vi "扭矩.vi"() -> ()   [LabVIEW 2020]
uses:
  <userlib>/DAQNavi Polymorphic VI/create/DAQNavi Create Channel(AI-Voltage).vi
  Global_Variable/Global.vi
  Global_Variable/A131258.vi
  <userlib>/DAQNavi Polymorphic VI/read/DAQNavi Read (Analog 1D DBL NChan 1Samp).vi
  <userlib>/_MGI/1D Array/MGI Running Average/MGI Running Average(DBL).vi
  <vilib>/ptbypt/NI_PtbyPt.lvlib
panel:
  out "左加载":dbl
  out "右加载":dbl
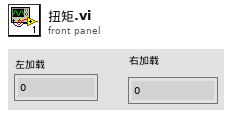
[diagram p1: front panel]
types:
  T1 = cluster{"左平均扭矩":cluster{"正转":dbl, "反转":dbl}, "左矩波动":cluster{"正转":dbl, "反转":dbl}, "左空载":cluster{"正转":dbl, "反转":dbl}, "右平均扭矩":cluster{"正转":dbl, "反转":dbl}, "右扭矩波动":cluster{"正转":dbl, "反转":dbl}, "右空载":cluster{"正转":dbl, "反转":dbl}, "扭矩对称":cluster{"左":dbl, "右":dbl}, "左零点漂移":cluster{"正":dbl, "反":dbl}, "右零点漂移":cluster{"正":dbl, "反":dbl}}
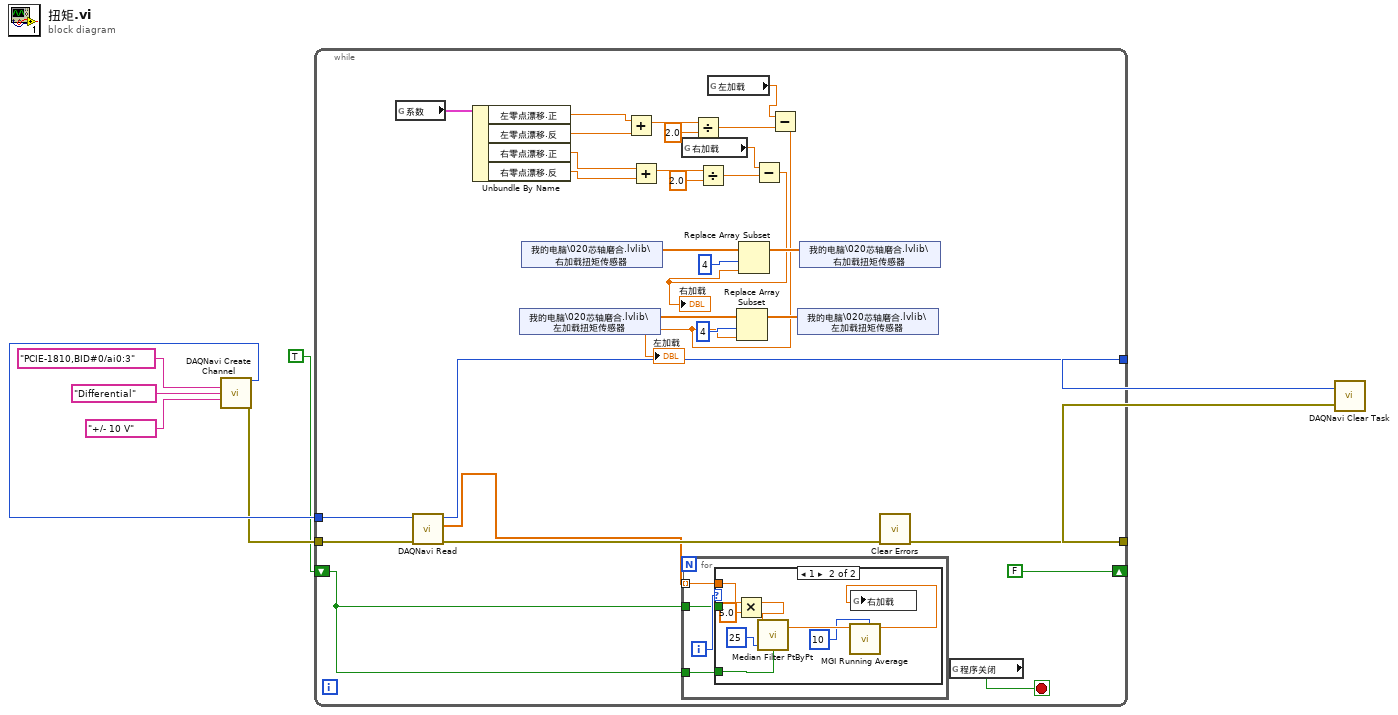
[diagram p0: block diagram]
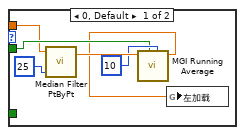
[diagram p2: hidden frame]
diagram:
  n1 = call-poly <userlib>:"DAQNavi Create Channel.vi"("physical channels"="PCIE-1810,BID#0/ai0:3", "signal type"="Differential", "value range"="+/- 10 V") -> ("task out"=w6:i32, "error out"=w5:errorcluster)  [unwired: 11 in]
  n2 = while {
    tunnel: w6 -> [w38]
    tunnel: w5 -> [w37]
    tunnel: [w33] -> w3
    tunnel: [w34] -> w2
    shift-right: [FALSE] -> _
    shift-left: TRUE -> [w9]
    stop <- w36 stop-if-true
    n3 = global read "A131258.vi" "系数"() -> (w24:T1)
    n4 = call-poly <userlib>:"DAQNavi Read.vi"("error in (no error)"=w37, "task in"=w38) -> ("error out"=w35:errorcluster, "data"=w25:dbl[], "task out"=w34:i32)  [unwired: 7 in]
    n5 = Unbundle By Name(w24) -> ("左零点漂移.正"=w23:dbl, "左零点漂移.反"=w22:dbl, "右零点漂移.正"=w14:dbl, "右零点漂移.反"=w13:dbl)
    n6 = shared-variable "我的电脑\\020芯轴磨合.lvlib\\左加载扭矩传感器"() -> (w27:sgl[])  [unwired: 1 in, 1 out]
    n7 = shared-variable "我的电脑\\020芯轴磨合.lvlib\\右加载扭矩传感器"() -> (w29:sgl[])  [unwired: 1 in, 1 out]
    n8 = Add(x=w23, y=w22) -> (x+y=w21:dbl)
    n9 = Add(x=w14, y=w13) -> (x+y=w15:dbl)
    n10 = global read "全局2.vi" "右加载"() -> (w11:dbl)
    n11 = for {
      tunnel: w25 -> [w41] mode=indexing
      tunnel: w9 -> [w40]
      tunnel: w9 -> [w39]
      i -> [w42]
      n12 = case shown="1" w42 {
        tunnel: w41 -> [w44 w55]
        tunnel: w40 -> [w46 _]
        tunnel: w39 -> [_ w52]
        frame 0, Default {
          n13 = call <vilib>:"Median Filter PtByPt.vi"("rank"=25, "x"=w44) -> ("Filtered x"=w48:dbl)  [unwired: 2 in, 1 out]
          n14 = call-poly <userlib>:"MGI Running Average.vi"("Averaging Size"=10, "Initialize? (F)"=w46, "Value"=w48) -> ("Average"=w43:dbl)  [unwired: 8 in]
          n15 = global write "全局1.vi" "左加载"(w43) -> ()
        }
        frame 1 {
          n16 = Multiply(x=w55, y=5.0) -> (x*y=w50:dbl)
          n17 = call <vilib>:"Median Filter PtByPt.vi"("initialize"=w52, "rank"=25, "x"=w50) -> ("Filtered x"=w54:dbl)  [unwired: 1 in, 1 out]
          n18 = call-poly <userlib>:"MGI Running Average.vi"("Averaging Size"=10, "Value"=w54) -> ("Average"=w49:dbl)  [unwired: 9 in]
          n19 = global write "全局2.vi" "右加载"(w49) -> ()
        }
      }
    }
    n20 = Divide(x=w21, y=2.0) -> (x/y=w19:dbl)
    n21 = Divide(x=w15, y=2.0) -> (x/y=w12:dbl)
    n22 = global read "全局1.vi" "左加载"() -> (w18:dbl)
    n23 = Subtract(x=w11, y=w12) -> (x-y=w10:dbl)
    "右加载" <- w10
    n24 = Replace Array Subset(array=w29, new element=w10, index=4 ("索引")) -> (w28:sgl[])
    n25 = Subtract(x=w18, y=w19) -> (x-y=w17:dbl)
    "左加载" <- w17
    n26 = Replace Array Subset(array=w27, new element=w17, index=4 ("索引")) -> (w26:sgl[])
    n27 = shared-variable "我的电脑\\020芯轴磨合.lvlib\\左加载扭矩传感器"(w26) -> ()  [unwired: 1 in, 1 out]
    n28 = shared-variable "我的电脑\\020芯轴磨合.lvlib\\右加载扭矩传感器"(w28) -> ()  [unwired: 1 in, 1 out]
    n29 = call <vilib>:"Clear Errors.vi"("error in (no error)"=w35) -> ("error out"=w33:errorcluster)  [unwired: 5 in, 1 out]
    n30 = global read "Global.vi" "程序关闭"() -> (w36:bool)
  }
  n31 = call <userlib>:"DAQNavi Clear Task.vi"("error in (no error)"=w3, "task in"=w2) -> ()  [unwired: 1 in, 1 out]
